vi "水样测试.vi"(11 "数据标记表":string(combo)="N") -> ()   [LabVIEW 2016, in "斯坦道多参数.lvlib"]
panel:
  out "运行状态":u16(ring) items=["空闲", "水样测试", "标样核查"]
  out "多参数运行日志":string
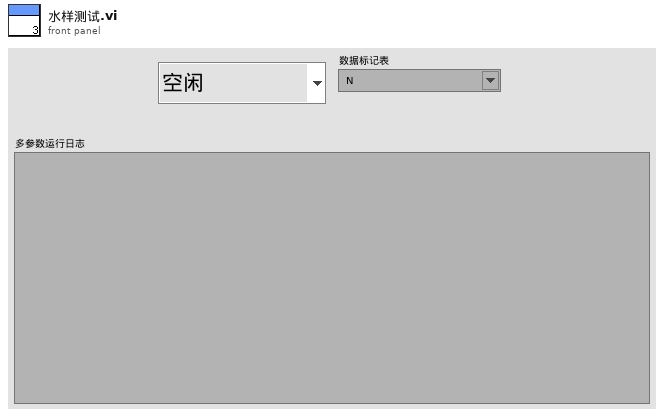
[diagram p1: front panel]
types:
  T1 = typedef "集成多参数单参数字段定义.ctl" = cluster{"时间":timestamp, "测量模式":string, "数据类型":string, "检测值":sgl, "单位":string, "数据标识":string, "信号值":sgl, "标样参考值":sgl, "因子编码":string, "探头温度":sgl, "LastTime":timestamp}
  T2 = cluster{"水温":bool, "pH":bool, "DO":bool, "DOper":bool, "电导率":bool, "ORP":bool, "浊度":bool, "叶绿素a":bool, "藻密度":bool, "COD":bool, "DO2":bool, "DOper":bool, "氯化物":bool, "氨氮":bool, "水中油":bool, "悬浮物":bool, "余氯":bool}
  T3 = cluster{"ph":bool, "DO":bool, "Cond":bool, "Turb":bool, "叶绿素a":bool, "藻密度":bool, "ORP":bool, "cod":bool, "DO2":bool, "氯化物":bool, "氨氮":bool, "水中油":bool, "悬浮物":bool, "余氯":bool}
  T4 = cluster{"温度测量值":sgl, "测量值":sgl, "温度偏移修正值":sgl, "信号值":sgl, "数据标识":string}
  T5 = cluster{"温度测量值":sgl, "DO%":sgl, "DOmg/L":sgl, "温度偏移修正值":sgl, "数据标识mg/L":string, "数据标识%":string}
  T6 = cluster{"CH":u16, "监测值":dbl, "信号值":sgl, "数据标识":string}
  T7 = cluster{"水样数据时间":timestamp, "水温":dbl, "pH":dbl, "DO":dbl, "DOper":dbl, "电导率":dbl, "ORP":dbl, "浊度":dbl, "叶绿素a":dbl, "藻密度":dbl, "COD":dbl, "DO2":dbl, "DO2per":dbl, "氯化物":dbl, "氨氮":dbl, "水中油":dbl, "悬浮物":dbl, "余氯":dbl}
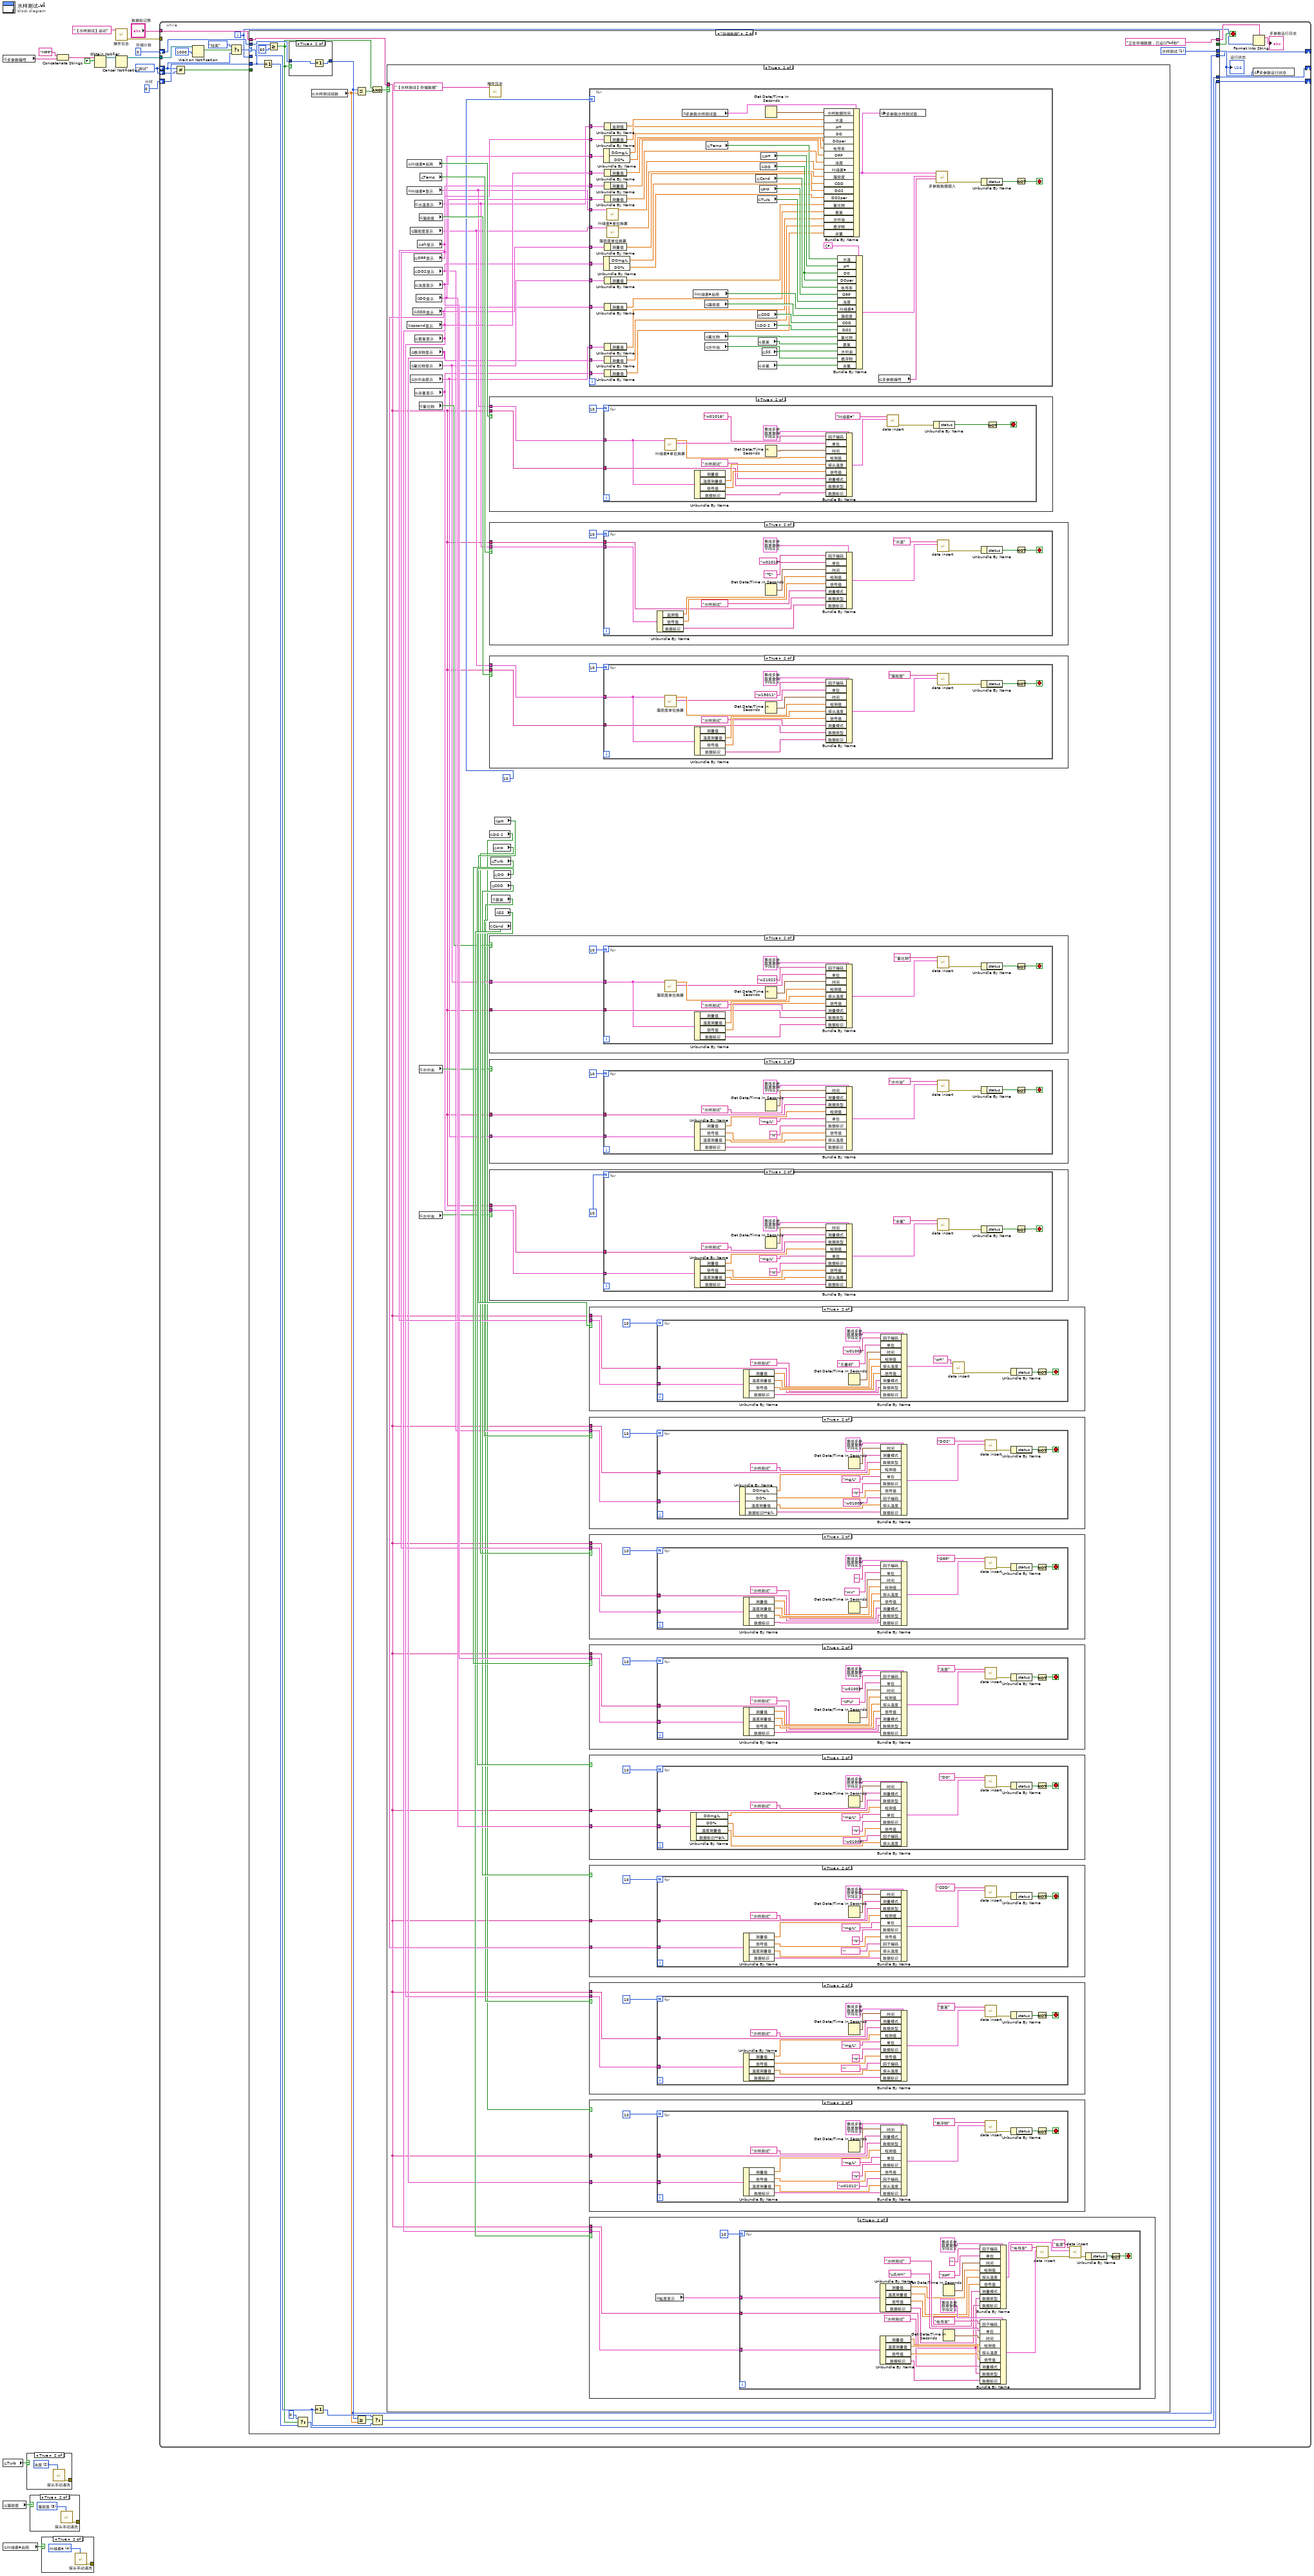
[diagram p0: block diagram]
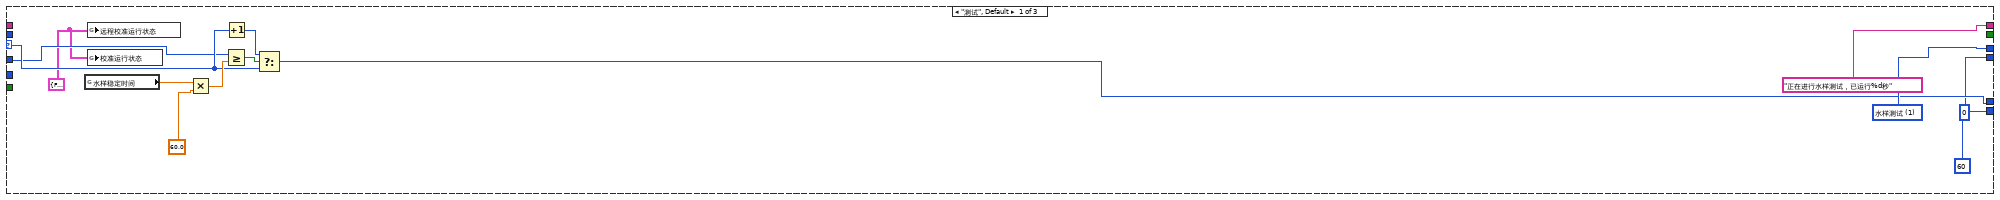
[diagram p5: hidden frame]
diagram:
  w7 = 0  # 存储计数
  w8 = 0  # 计时
  w3 = enum16{"测试", "存储数据", "结束"}."测试" ("枚举")
  n1 = global read "多参数全局变量.vi" "多参数编号"() -> (w9:string)
  n2 = global read "断电保存变量.vi" "Turb"() -> (w6:bool)
  n3 = global read "断电保存变量.vi" "藻密度"() -> (w4:bool)
  n4 = global read "断电保存变量.vi" "叶绿素a启用"() -> (w5:bool)
  n5 = case shown="True" w6 {
    tunnel: [_ w16] -> _
    frame False {
    }
    frame True {
      w17 = u16 2 items=["pH", "DO", "浊度", "电导率", "叶绿素a", "藻密度", "ORP", "DO2"] ("校准参数")
      n6 = call "探头手动清洗.vi"("校准参数"=w17) -> ("error out"=w16:errorcluster)  [unwired: 10 in]
    }
  }
  n7 = case shown="True" w4 {
    tunnel: [_ w18] -> _
    frame False {
    }
    frame True {
      w19 = u16 5 items=["pH", "DO", "浊度", "电导率", "叶绿素a", "藻密度", "ORP", "DO2"] ("校准参数")
      n8 = call "探头手动清洗.vi"("校准参数"=w19) -> ("error out"=w18:errorcluster)  [unwired: 10 in]
    }
  }
  n9 = case shown="True" w5 {
    tunnel: [_ w20] -> _
    frame False {
    }
    frame True {
      w21 = u16 4 items=["pH", "DO", "浊度", "电导率", "叶绿素a", "藻密度", "ORP", "DO2"] ("校准参数")
      n10 = call "探头手动清洗.vi"("校准参数"=w21) -> ("error out"=w20:errorcluster)  [unwired: 10 in]
    }
  }
  n11 = Concatenate Strings("MPP" ("名称（未命名）"), w9) -> (w10:string)
  n12 = Obtain Notifier(name (unnamed)=w10, notification data type=FALSE) -> (notifier out=w13:refnum<notifier>)  [unwired: 2 in, 2 out]
  n13 = call "操作日志.vi"("日志信息"="【水样测试】启动") -> ("error out"=w1:errorcluster)  [unwired: 10 in]
  n14 = Cancel Notification(0:w13) -> (8:w12:refnum<notifier>)  [unwired: 1 in, 2 out]
  n15 = while {
    shift-right: [w26] -> _
    shift-left: w3 -> [w24]
    tunnel: w12 -> [w37]
    tunnel: "数据标记表" -> [w32]
    shift-right: [w28] -> _
    shift-left: w8 -> [w30]
    shift-right: [w27] -> _
    shift-left: w7 -> [w29]
    shift-left: w3 -> [w23]
    tunnel: w1 -> [_]
    i -> [w25]
    stop <- w40 stop-if-true
    n16 = Not Equal?(x=w24, y=w23) -> (x != y?=w22:bool)
    n17 = Wait on Notification(notifier=w37, timeout in ms (-1)=1000 ("超时毫秒(-1)")) -> (notification=w35:bool)  [unwired: 2 in, 3 out]
    n18 = Select(t=enum16{"测试", "存储数据", "结束"}."结束" ("枚举"), s=w35, f=w24) -> (s? t:f=w33:enum16{"测试", "存储数据", "结束"})
    n19 = case shown="\"存储数据\"" w33 {
      selector: w33 -> [w47 w61 _]
      tunnel: [_ _ TRUE] -> w40
      tunnel: ["正在进行水样测试，已运行%d秒" ("格式字符串") "正在存储数据，已运行%d秒" ("格式字符串") "测试停止，累计运行%d秒" ("格式字符串")] -> w39
      tunnel: [w52 w66 w470] -> w31
      tunnel: w32 -> [_ w71 _]
      tunnel: w30 -> [_ w69 _]
      tunnel: w29 -> [_ w70 _]
      tunnel: [60 w54 0] -> w28
      tunnel: [0 w60 0] -> w27
      tunnel: [w45 w64 enum16{"测试", "存储数据", "结束"}."结束" ("枚举")] -> w26
      tunnel: w25 -> [w42 _ _]
      tunnel: w22 -> [_ _ w466]
      frame "测试", Default {
        w41 = T3 {"ph"=FALSE, "DO"=FALSE, "Cond"=FALSE, "Turb"=FALSE, "叶绿素a"=FALSE, "藻密度"=FALSE, "ORP"=FALSE, "cod"=FALSE, "DO2"=FALSE, "氯化物"=FALSE, "氨氮"=FALSE, "水中油"=FALSE, "悬浮物"=FALSE, "余氯"=FALSE} ("远程校准运行状态")
        w52 = u16 1 items=["空闲", "水样测试", "标样核查"] ("多参数运行状态")
        n20 = global read "断电保存变量.vi" "水样稳定时间"() -> (w51:dbl)
        n21 = global write "多参数全局变量.vi" "远程校准运行状态"(w41) -> ()
        n22 = global write "多参数全局变量.vi" "校准运行状态"(w41) -> ()
        n23 = Multiply(x=w51, y=60.0) -> (x*y=w49:dbl)
        n24 = Greater Or Equal?(x=w42, y=w49) -> (x >= y?=w48:bool)
        n25 = Increment(x=w47) -> (x+1=w46:enum16{"测试", "存储数据", "结束"})
        n26 = Select(t=w46, s=w48, f=w47) -> (s? t:f=w45:enum16{"测试", "存储数据", "结束"})
      }
      frame "存储数据" {
        w66 = u16 1 items=["空闲", "水样测试", "标样核查"] ("多参数运行状态")
        n27 = Increment(x=w69) -> (x+1=w56:i32)
        n28 = Greater Or Equal?(x=w69, y=60) -> (x >= y?=w57:bool)
        n29 = case shown="True" w57 {
          tunnel: w70 -> [w72 w74]
          tunnel: [w72 w73] -> w60
          frame False {
          }
          frame True {
            n30 = Increment(x=w74) -> (x+1=w73:i32)
          }
        }
        n31 = Select(t=0, s=w57, f=w56) -> (s? t:f=w54:i32)
        n32 = global read "断电保存变量.vi" "水样测试组数"() -> (w59:dbl)
        n33 = Increment(x=w61) -> (x+1=w62:enum16{"测试", "存储数据", "结束"})
        n34 = Less Or Equal?(x=w60, y=w59) -> (x <= y?=w65:bool)
        n35 = Greater Or Equal?(x=w60, y=w59) -> (x >= y?=w58:bool)
        n36 = And(x=w57, y=w65) -> (x .and. y?=w63:bool)
        n37 = Select(t=w62, s=w58, f=w61) -> (s? t:f=w64:enum16{"测试", "存储数据", "结束"})
        n38 = case shown="True" w63 {
          tunnel: w71 -> [_ w75]
          frame False {
          }
          frame True {
            n39 = global read "断电保存变量.vi" "叶绿素a启用"() -> (w107:bool)
            n40 = global read "多参数全局变量.vi" "叶绿素a显示"() -> (w92:T4)
            n41 = global read "多参数全局变量.vi" "spcond显示"() -> (w98:T4)
            n42 = global read "多参数全局变量.vi" "藻密度显示"() -> (w94:T4)
            n43 = global read "多参数全局变量.vi" "悬浮物显示"() -> (w79:T4)
            n44 = global read "多参数全局变量.vi" "氯化物显示"() -> (w84:T4)
            n45 = global read "多参数全局变量.vi" "水中油显示"() -> (w80:T4)
            n46 = global read "多参数全局变量.vi" "COD显示"() -> (w89:T4)
            n47 = global read "多参数全局变量.vi" "ORP显示"() -> (w91:T4)
            n48 = global read "多参数全局变量.vi" "DO2显示"() -> (w86:T5)
            n49 = global read "多参数全局变量.vi" "水温显示"() -> (w93:T6)
            n50 = global read "多参数全局变量.vi" "浊度显示"() -> (w96:T4)
            n51 = global read "多参数全局变量.vi" "氨氮显示"() -> (w82:T4)
            n52 = global read "多参数全局变量.vi" "余氯显示"() -> (w76:T4)
            n53 = global read "多参数全局变量.vi" "DO显示"() -> (w95:T5)
            n54 = global read "多参数全局变量.vi" "ph显示"() -> (w97:T4)
            n55 = global read "断电保存变量.vi" "藻密度"() -> (w101:bool)
            n56 = global read "断电保存变量.vi" "氯化物"() -> (w85:bool)
            n57 = global read "断电保存变量.vi" "水中油"() -> (w81:bool)
            n58 = global read "断电保存变量.vi" "水中油"() -> (w77:bool)
            n59 = global read "断电保存变量.vi" "Temp"() -> (w102:bool)
            n60 = call "操作日志.vi"("日志信息"="【水样测试】存储数据") -> ()  [unwired: 10 in, 1 out]
            n61 = case shown="True" w107 {
              tunnel: w75 -> [_ w341]
              tunnel: w92 -> [_ w339]
              frame False {
              }
              frame True {
                n62 = for {
                  N: 10 -> [_]
                  tunnel: w341 -> [w347]
                  tunnel: w339 -> [w344]
                  stop <- w351 stop-if-true
                  n63 = call "叶绿素a单位换算.vi"("叶绿素a显示"=w344) -> ("检测值1.单位"=w343:string, "测量值"=w342:sgl)  [unwired: 8 in, 1 out]
                  n64 = Unbundle By Name(w344) -> ("温度测量值"=w357:sgl, "信号值"=w350:sgl, "数据标识"=w346:string)  [unwired: 1 out]
                  n65 = Get Date/Time In Seconds() -> (seconds since 1Jan1904=w349:timestamp)
                  n66 = Bundle By Name(cluster=T1 {"时间"=timestamp(0 s since 1904-01-01), "测量模式"="水样测试", "数据类型"="N", "检测值"=0.0, "单位"="mg/L", "数据标识"="N", "信号值"=0.0, "标样参考值"=0.0, "因子编码"="", "探头温度"=0.0, "LastTime"=timestamp(0 s since 1904-01-01)} ("data"), "因子编码"="w01016", "单位"=w343, "时间"=w349, "检测值"=w342, "探头温度"=w357, "信号值"=w350, "测量模式"="水样测试", "数据类型"=w347, "数据标识"=w346) -> (w355:T1)
                  n67 = call "data insert.vi"("data"=w355, "table in"="叶绿素a" ("table输入")) -> ("error out"=w353:errorcluster)  [unwired: 9 in]
                  n68 = Unbundle By Name(w353) -> ("status"=w352:bool)
                  n69 = Not(x=w352) -> (.not. x?=w351:bool)
                }
              }
            }
            n70 = case shown="True" w102 {
              tunnel: w75 -> [_ w450]
              tunnel: w93 -> [_ w448]
              frame False {
              }
              frame True {
                n71 = for {
                  N: 10 -> [_]
                  tunnel: w450 -> [w454]
                  tunnel: w448 -> [w453]
                  stop <- w458 stop-if-true
                  n72 = Unbundle By Name(w453) -> ("监测值"=w461:dbl, "信号值"=w456:sgl, "数据标识"=w452:string)
                  n73 = Get Date/Time In Seconds() -> (seconds since 1Jan1904=w457:timestamp)
                  n74 = Bundle By Name(cluster=T1 {"时间"=timestamp(0 s since 1904-01-01), "测量模式"="水样测试", "数据类型"="N", "检测值"=0.0, "单位"="mg/L", "数据标识"="N", "信号值"=0.0, "标样参考值"=0.0, "因子编码"="", "探头温度"=0.0, "LastTime"=timestamp(0 s since 1904-01-01)} ("data"), "因子编码"="w01010", "单位"="℃", "时间"=w457, "检测值"=w461, "信号值"=w456, "测量模式"="水样测试", "数据类型"=w454, "数据标识"=w452) -> (w464:T1)
                  n75 = call "data insert.vi"("data"=w464, "table in"="水温" ("table输入")) -> ("error out"=w460:errorcluster)  [unwired: 9 in]
                  n76 = Unbundle By Name(w460) -> ("status"=w459:bool)
                  n77 = Not(x=w459) -> (.not. x?=w458:bool)
                }
              }
            }
            n78 = case shown="True" w101 {
              tunnel: w75 -> [_ w322]
              tunnel: w94 -> [_ w320]
              frame False {
              }
              frame True {
                n79 = for {
                  N: 10 -> [_]
                  tunnel: w322 -> [w329]
                  tunnel: w320 -> [w325]
                  stop <- w330 stop-if-true
                  n80 = call "藻密度单位换算.vi"("藻密度显示"=w325) -> ("检测值1.单位"=w323:string, "测量值"=w324:sgl)  [unwired: 8 in, 1 out]
                  n81 = Unbundle By Name(w325) -> ("温度测量值"=w338:sgl, "信号值"=w331:sgl, "数据标识"=w327:string)  [unwired: 1 out]
                  n82 = Get Date/Time In Seconds() -> (seconds since 1Jan1904=w332:timestamp)
                  n83 = Bundle By Name(cluster=T1 {"时间"=timestamp(0 s since 1904-01-01), "测量模式"="水样测试", "数据类型"="N", "检测值"=0.0, "单位"="mg/L", "数据标识"="N", "信号值"=0.0, "标样参考值"=0.0, "因子编码"="", "探头温度"=0.0, "LastTime"=timestamp(0 s since 1904-01-01)} ("data"), "因子编码"="w19011", "单位"=w323, "时间"=w332, "检测值"=w324, "探头温度"=w338, "信号值"=w331, "测量模式"="水样测试", "数据类型"=w329, "数据标识"=w327) -> (w333:T1)
                  n84 = call "data insert.vi"("data"=w333, "table in"="藻密度" ("table输入")) -> ("error out"=w335:errorcluster)  [unwired: 9 in]
                  n85 = Unbundle By Name(w335) -> ("status"=w334:bool)
                  n86 = Not(x=w334) -> (.not. x?=w330:bool)
                }
              }
            }
            n87 = global read "断电保存变量.vi" "DO 2"() -> (w87:bool)
            n88 = global read "断电保存变量.vi" "Cond"() -> (w105:bool)
            n89 = case shown="True" w85 {
              tunnel: w75 -> [_ w188]
              tunnel: w84 -> [_ w186]
              frame False {
              }
              frame True {
                n90 = for {
                  N: 10 -> [_]
                  tunnel: w188 -> [w197]
                  tunnel: w186 -> [w193]
                  stop <- w198 stop-if-true
                  n91 = call "藻密度单位换算.vi"("藻密度显示"=w193) -> ("检测值1.单位"=w191:string, "测量值"=w192:sgl)  [unwired: 8 in, 1 out]
                  n92 = Unbundle By Name(w193) -> ("温度测量值"=w204:sgl, "信号值"=w199:sgl, "数据标识"=w195:string)  [unwired: 1 out]
                  n93 = Get Date/Time In Seconds() -> (seconds since 1Jan1904=w200:timestamp)
                  n94 = Bundle By Name(cluster=T1 {"时间"=timestamp(0 s since 1904-01-01), "测量模式"="水样测试", "数据类型"="N", "检测值"=0.0, "单位"="mg/L", "数据标识"="N", "信号值"=0.0, "标样参考值"=0.0, "因子编码"="", "探头温度"=0.0, "LastTime"=timestamp(0 s since 1904-01-01)} ("data"), "因子编码"="w21022", "单位"=w191, "时间"=w200, "检测值"=w192, "探头温度"=w204, "信号值"=w199, "测量模式"="水样测试", "数据类型"=w197, "数据标识"=w195) -> (w201:T1)
                  n95 = call "data insert.vi"("data"=w201, "table in"="氯化物") -> ("error out"=w203:errorcluster)  [unwired: 9 in]
                  n96 = Unbundle By Name(w203) -> ("status"=w202:bool)
                  n97 = Not(x=w202) -> (.not. x?=w198:bool)
                }
              }
            }
            n98 = case shown="True" w81 {
              tunnel: w75 -> [_ w149]
              tunnel: w80 -> [_ w147]
              frame False {
              }
              frame True {
                n99 = for {
                  N: 10 -> [_]
                  tunnel: w149 -> [w162]
                  tunnel: w147 -> [w155]
                  stop <- w165 stop-if-true
                  n100 = Unbundle By Name(w155) -> ("测量值"=w154:sgl, "信号值"=w153:sgl, "温度测量值"=w152:sgl, "数据标识"=w151:string)
                  n101 = Get Date/Time In Seconds() -> (seconds since 1Jan1904=w164:timestamp)
                  n102 = Bundle By Name(cluster=T1 {"时间"=timestamp(0 s since 1904-01-01), "测量模式"="水样测试", "数据类型"="N", "检测值"=0.0, "单位"="mg/L", "数据标识"="N", "信号值"=0.0, "标样参考值"=0.0, "因子编码"="", "探头温度"=0.0, "LastTime"=timestamp(0 s since 1904-01-01)} ("data"), "时间"=w164, "测量模式"="水样测试", "数据类型"=w162, "检测值"=w154, "单位"="mg/L", "数据标识"="N" ("水样数据标识"), "信号值"=w153, "探头温度"=w152, "数据标识"=w151) -> (w157:T1)
                  n103 = call "data insert.vi"("data"=w157, "table in"="水中油") -> ("error out"=w158:errorcluster)  [unwired: 9 in]
                  n104 = Unbundle By Name(w158) -> ("status"=w159:bool)
                  n105 = Not(x=w159) -> (.not. x?=w165:bool)
                }
              }
            }
            n106 = case shown="True" w77 {
              tunnel: w75 -> [_ w110]
              tunnel: w76 -> [_ w108]
              frame False {
              }
              frame True {
                n107 = for {
                  N: 10 -> [_]
                  tunnel: w110 -> [w123]
                  tunnel: w108 -> [w116]
                  stop <- w126 stop-if-true
                  n108 = Unbundle By Name(w116) -> ("测量值"=w115:sgl, "信号值"=w114:sgl, "温度测量值"=w113:sgl, "数据标识"=w112:string)
                  n109 = Get Date/Time In Seconds() -> (seconds since 1Jan1904=w125:timestamp)
                  n110 = Bundle By Name(cluster=T1 {"时间"=timestamp(0 s since 1904-01-01), "测量模式"="水样测试", "数据类型"="N", "检测值"=0.0, "单位"="mg/L", "数据标识"="N", "信号值"=0.0, "标样参考值"=0.0, "因子编码"="", "探头温度"=0.0, "LastTime"=timestamp(0 s since 1904-01-01)} ("data"), "时间"=w125, "测量模式"="水样测试", "数据类型"=w123, "检测值"=w115, "单位"="mg/L", "数据标识"="N" ("水样数据标识"), "信号值"=w114, "探头温度"=w113, "数据标识"=w112) -> (w118:T1)
                  n111 = call "data insert.vi"("data"=w118, "table in"="余氯") -> ("error out"=w119:errorcluster)  [unwired: 9 in]
                  n112 = Unbundle By Name(w119) -> ("status"=w120:bool)
                  n113 = Not(x=w120) -> (.not. x?=w126:bool)
                }
              }
            }
            n114 = global read "断电保存变量.vi" "Turb"() -> (w106:bool)
            n115 = global read "断电保存变量.vi" "COD"() -> (w88:bool)
            n116 = global read "断电保存变量.vi" "氨氮"() -> (w83:bool)
            n117 = global read "断电保存变量.vi" "orp"() -> (w100:bool)
            n118 = global read "断电保存变量.vi" "DO"() -> (w104:bool)
            n119 = global read "断电保存变量.vi" "pH"() -> (w103:bool)
            n120 = global read "断电保存变量.vi" "SS"() -> (w78:bool)
            n121 = for {
              N: 10 -> [_]
              tunnel: w93 -> [w280]
              tunnel: w97 -> [w279]
              tunnel: w95 -> [w278]
              tunnel: w98 -> [w277]
              tunnel: w91 -> [w276]
              tunnel: w96 -> [w275]
              tunnel: w92 -> [w265]
              tunnel: w94 -> [w267]
              tunnel: w89 -> [w273]
              tunnel: w86 -> [w270]
              tunnel: w84 -> [w261]
              tunnel: w82 -> [w259]
              tunnel: w80 -> [w252]
              tunnel: w79 -> [w249]
              tunnel: w76 -> [w246]
              stop <- w282 stop-if-true
              n122 = Unbundle By Name(w278) -> ("DOmg/L"=w297:sgl, "DO%"=w296:sgl)
              n123 = Unbundle By Name(w270) -> ("DOmg/L"=w269:sgl, "DO%"=w268:sgl)
              n124 = Unbundle By Name(w280) -> ("监测值"=w299:dbl)
              n125 = Unbundle By Name(w279) -> ("测量值"=w298:sgl)
              n126 = Unbundle By Name(w277) -> ("测量值"=w295:sgl)
              n127 = Unbundle By Name(w276) -> ("测量值"=w294:sgl)
              n128 = Unbundle By Name(w275) -> ("测量值"=w293:sgl)
              n129 = Unbundle By Name(w273) -> ("测量值"=w272:sgl)
              n130 = Unbundle By Name(w261) -> ("测量值"=w260:sgl)
              n131 = Unbundle By Name(w259) -> ("测量值"=w258:sgl)
              n132 = Unbundle By Name(w252) -> ("测量值"=w251:sgl)
              n133 = Unbundle By Name(w249) -> ("测量值"=w248:sgl)
              n134 = Unbundle By Name(w246) -> ("测量值"=w245:sgl)
              n135 = call "叶绿素a单位换算.vi"("叶绿素a显示"=w265) -> ("测量值"=w264:sgl)  [unwired: 8 in, 2 out]
              n136 = call "藻密度单位换算.vi"("藻密度显示"=w267) -> ("测量值"=w266:sgl)  [unwired: 8 in, 2 out]
              n137 = global read "多参数全局变量.vi" "多参数水样测试值"() -> (w256:T7)
              n138 = global read "断电保存变量.vi" "叶绿素a启用"() -> (w286:bool)
              n139 = global read "断电保存变量.vi" "藻密度"() -> (w289:bool)
              n140 = global read "断电保存变量.vi" "氯化物"() -> (w262:bool)
              n141 = global read "断电保存变量.vi" "水中油"() -> (w253:bool)
              n142 = global read "断电保存变量.vi" "Temp"() -> (w288:bool)
              n143 = global read "断电保存变量.vi" "Cond"() -> (w291:bool)
              n144 = global read "断电保存变量.vi" "DO 2"() -> (w271:bool)
              n145 = global read "断电保存变量.vi" "Turb"() -> (w290:bool)
              n146 = global read "断电保存变量.vi" "COD"() -> (w274:bool)
              n147 = global read "断电保存变量.vi" "氨氮"() -> (w257:bool)
              n148 = global read "断电保存变量.vi" "余氯"() -> (w247:bool)
              n149 = global read "断电保存变量.vi" "orp"() -> (w287:bool)
              n150 = global read "断电保存变量.vi" "DO"() -> (w285:bool)
              n151 = global read "断电保存变量.vi" "pH"() -> (w292:bool)
              n152 = global read "断电保存变量.vi" "SS"() -> (w250:bool)
              n153 = Get Date/Time In Seconds() -> (seconds since 1Jan1904=w300:timestamp)
              n154 = Bundle By Name(cluster=w256, "水样数据时间"=w300, "水温"=w299, "pH"=w298, "DO"=w297, "DOper"=w296, "电导率"=w295, "ORP"=w294, "浊度"=w293, "叶绿素a"=w264, "藻密度"=w266, "COD"=w272, "DO2"=w269, "DO2per"=w268, "氯化物"=w260, "氨氮"=w258, "水中油"=w251, "悬浮物"=w248, "余氯"=w245) -> (w263:T7)
              n155 = Bundle By Name(cluster=T2 {"水温"=FALSE, "pH"=FALSE, "DO"=FALSE, "DOper"=FALSE, "电导率"=FALSE, "ORP"=FALSE, "浊度"=FALSE, "叶绿素a"=FALSE, "藻密度"=FALSE, "COD"=FALSE, "DO2"=FALSE, "DOper"=FALSE, "氯化物"=FALSE, "氨氮"=FALSE, "水中油"=FALSE, "悬浮物"=FALSE, "余氯"=FALSE} ("columns enable"), "水温"=w288, "pH"=w292, "DO"=w285, "DOper"=w285, "电导率"=w291, "ORP"=w287, "浊度"=w290, "叶绿素a"=w286, "藻密度"=w289, "COD"=w274, "DO2"=w271, "氯化物"=w262, "氨氮"=w257, "水中油"=w253, "悬浮物"=w250, "余氯"=w247) -> (w254:T2)
              n156 = global read "多参数全局变量.vi" "多参数编号"() -> (w281:string)
              n157 = global write "多参数全局变量.vi" "多参数水样测试值"(w263) -> ()
              n158 = call "多参数数据插入.vi"("编号"=w281, "columns enable"=w254, "data in"=w263) -> ("error out"=w284:errorcluster)  [unwired: 8 in]
              n159 = Unbundle By Name(w284) -> ("status"=w283:bool)
              n160 = Not(x=w283) -> (.not. x?=w282:bool)
            }
            n161 = case shown="True" w103 {
              tunnel: w75 -> [_ w431]
              tunnel: w97 -> [_ w429]
              frame False {
              }
              frame True {
                n162 = for {
                  N: 10 -> [_]
                  tunnel: w431 -> [w435]
                  tunnel: w429 -> [w434]
                  stop <- w439 stop-if-true
                  n163 = Unbundle By Name(w434) -> ("测量值"=w443:sgl, "温度测量值"=w442:sgl, "信号值"=w437:sgl, "数据标识"=w433:string)
                  n164 = Get Date/Time In Seconds() -> (seconds since 1Jan1904=w438:timestamp)
                  n165 = Bundle By Name(cluster=T1 {"时间"=timestamp(0 s since 1904-01-01), "测量模式"="水样测试", "数据类型"="N", "检测值"=0.0, "单位"="mg/L", "数据标识"="N", "信号值"=0.0, "标样参考值"=0.0, "因子编码"="", "探头温度"=0.0, "LastTime"=timestamp(0 s since 1904-01-01)} ("data"), "因子编码"="w01001", "单位"="无量纲", "时间"=w438, "检测值"=w443, "探头温度"=w442, "信号值"=w437, "测量模式"="水样测试", "数据类型"=w435, "数据标识"=w433) -> (w447:T1)
                  n166 = call "data insert.vi"("data"=w447, "table in"="pH" ("table输入")) -> ("error out"=w441:errorcluster)  [unwired: 9 in]
                  n167 = Unbundle By Name(w441) -> ("status"=w440:bool)
                  n168 = Not(x=w440) -> (.not. x?=w439:bool)
                }
              }
            }
            n169 = case shown="True" w87 {
              tunnel: w75 -> [_ w207]
              tunnel: w86 -> [_ w205]
              frame False {
              }
              frame True {
                n170 = for {
                  N: 10 -> [_]
                  tunnel: w207 -> [w221]
                  tunnel: w205 -> [w211]
                  stop <- w224 stop-if-true
                  n171 = Unbundle By Name(w211) -> ("DOmg/L"=w220:sgl, "DO%"=w213:sgl, "温度测量值"=w214:sgl, "数据标识mg/L"=w210:string)
                  n172 = Get Date/Time In Seconds() -> (seconds since 1Jan1904=w223:timestamp)
                  n173 = Bundle By Name(cluster=T1 {"时间"=timestamp(0 s since 1904-01-01), "测量模式"="水样测试", "数据类型"="N", "检测值"=0.0, "单位"="mg/L", "数据标识"="N", "信号值"=0.0, "标样参考值"=0.0, "因子编码"="", "探头温度"=0.0, "LastTime"=timestamp(0 s since 1904-01-01)} ("data"), "时间"=w223, "测量模式"="水样测试", "数据类型"=w221, "检测值"=w220, "单位"="mg/L", "数据标识"="N" ("水样数据标识"), "信号值"=w213, "因子编码"="w01009", "探头温度"=w214, "数据标识"=w210) -> (w212:T1)
                  n174 = call "data insert.vi"("data"=w212, "table in"="DO2") -> ("error out"=w216:errorcluster)  [unwired: 9 in]
                  n175 = Unbundle By Name(w216) -> ("status"=w217:bool)
                  n176 = Not(x=w217) -> (.not. x?=w224:bool)
                }
              }
            }
            n177 = case shown="True" w100 {
              tunnel: w75 -> [_ w303]
              tunnel: w91 -> [_ w301]
              frame False {
              }
              frame True {
                n178 = for {
                  N: 10 -> [_]
                  tunnel: w303 -> [w309]
                  tunnel: w301 -> [w307]
                  stop <- w312 stop-if-true
                  n179 = Unbundle By Name(w307) -> ("测量值"=w319:sgl, "温度测量值"=w317:sgl, "信号值"=w310:sgl, "数据标识"=w306:string)
                  n180 = Get Date/Time In Seconds() -> (seconds since 1Jan1904=w311:timestamp)
                  n181 = Bundle By Name(cluster=T1 {"时间"=timestamp(0 s since 1904-01-01), "测量模式"="水样测试", "数据类型"="N", "检测值"=0.0, "单位"="mg/L", "数据标识"="N", "信号值"=0.0, "标样参考值"=0.0, "因子编码"="", "探头温度"=0.0, "LastTime"=timestamp(0 s since 1904-01-01)} ("data"), "因子编码"="", "单位"="mV", "时间"=w311, "检测值"=w319, "探头温度"=w317, "信号值"=w310, "测量模式"="水样测试", "数据类型"=w309, "数据标识"=w306) -> (w304:T1)
                  n182 = call "data insert.vi"("data"=w304, "table in"="ORP" ("table输入")) -> ("error out"=w315:errorcluster)  [unwired: 9 in]
                  n183 = Unbundle By Name(w315) -> ("status"=w314:bool)
                  n184 = Not(x=w314) -> (.not. x?=w312:bool)
                }
              }
            }
            n185 = case shown="True" w106 {
              tunnel: w75 -> [_ w360]
              tunnel: w96 -> [_ w358]
              frame False {
              }
              frame True {
                n186 = for {
                  N: 10 -> [_]
                  tunnel: w360 -> [w364]
                  tunnel: w358 -> [w363]
                  stop <- w368 stop-if-true
                  n187 = Unbundle By Name(w363) -> ("测量值"=w372:sgl, "温度测量值"=w371:sgl, "信号值"=w366:sgl, "数据标识"=w362:string)
                  n188 = Get Date/Time In Seconds() -> (seconds since 1Jan1904=w367:timestamp)
                  n189 = Bundle By Name(cluster=T1 {"时间"=timestamp(0 s since 1904-01-01), "测量模式"="水样测试", "数据类型"="N", "检测值"=0.0, "单位"="mg/L", "数据标识"="N", "信号值"=0.0, "标样参考值"=0.0, "因子编码"="", "探头温度"=0.0, "LastTime"=timestamp(0 s since 1904-01-01)} ("data"), "因子编码"="w01003", "单位"="NTU", "时间"=w367, "检测值"=w372, "探头温度"=w371, "信号值"=w366, "测量模式"="水样测试", "数据类型"=w364, "数据标识"=w362) -> (w375:T1)
                  n190 = call "data insert.vi"("data"=w375, "table in"="浊度" ("table输入")) -> ("error out"=w370:errorcluster)  [unwired: 9 in]
                  n191 = Unbundle By Name(w370) -> ("status"=w369:bool)
                  n192 = Not(x=w369) -> (.not. x?=w368:bool)
                }
              }
            }
            n193 = case shown="True" w104 {
              tunnel: w75 -> [_ w412]
              tunnel: w95 -> [_ w410]
              frame False {
              }
              frame True {
                n194 = for {
                  N: 10 -> [_]
                  tunnel: w412 -> [w424]
                  tunnel: w410 -> [w415]
                  stop <- w428 stop-if-true
                  n195 = Unbundle By Name(w415) -> ("DOmg/L"=w423:sgl, "DO%"=w417:sgl, "温度测量值"=w418:sgl)  [unwired: 1 out]
                  n196 = Get Date/Time In Seconds() -> (seconds since 1Jan1904=w426:timestamp)
                  n197 = Bundle By Name(cluster=T1 {"时间"=timestamp(0 s since 1904-01-01), "测量模式"="水样测试", "数据类型"="N", "检测值"=0.0, "单位"="mg/L", "数据标识"="N", "信号值"=0.0, "标样参考值"=0.0, "因子编码"="", "探头温度"=0.0, "LastTime"=timestamp(0 s since 1904-01-01)} ("data"), "时间"=w426, "测量模式"="水样测试", "数据类型"=w424, "检测值"=w423, "单位"="mg/L", "数据标识"="N", "信号值"=w417, "因子编码"="w01009", "探头温度"=w418) -> (w416:T1)
                  n198 = call "data insert.vi"("data"=w416, "table in"="DO") -> ("error out"=w420:errorcluster)  [unwired: 9 in]
                  n199 = Unbundle By Name(w420) -> ("status"=w421:bool)
                  n200 = Not(x=w421) -> (.not. x?=w428:bool)
                }
              }
            }
            n201 = case shown="True" w88 {
              tunnel: w75 -> [_ w227]
              tunnel: w89 -> [_ w225]
              frame False {
              }
              frame True {
                n202 = for {
                  N: 10 -> [_]
                  tunnel: w227 -> [w240]
                  tunnel: w225 -> [w230]
                  stop <- w244 stop-if-true
                  n203 = Unbundle By Name(w230) -> ("测量值"=w239:sgl, "信号值"=w232:sgl, "温度测量值"=w233:sgl, "数据标识"=w229:string)
                  n204 = Get Date/Time In Seconds() -> (seconds since 1Jan1904=w242:timestamp)
                  n205 = Bundle By Name(cluster=T1 {"时间"=timestamp(0 s since 1904-01-01), "测量模式"="水样测试", "数据类型"="N", "检测值"=0.0, "单位"="mg/L", "数据标识"="N", "信号值"=0.0, "标样参考值"=0.0, "因子编码"="", "探头温度"=0.0, "LastTime"=timestamp(0 s since 1904-01-01)} ("data"), "时间"=w242, "测量模式"="水样测试", "数据类型"=w240, "检测值"=w239, "单位"="mg/L", "数据标识"="N" ("水样数据标识"), "信号值"=w232, "因子编码"="", "探头温度"=w233, "数据标识"=w229) -> (w231:T1)
                  n206 = call "data insert.vi"("data"=w231, "table in"="COD") -> ("error out"=w235:errorcluster)  [unwired: 9 in]
                  n207 = Unbundle By Name(w235) -> ("status"=w236:bool)
                  n208 = Not(x=w236) -> (.not. x?=w244:bool)
                }
              }
            }
            n209 = case shown="True" w83 {
              tunnel: w75 -> [_ w168]
              tunnel: w82 -> [_ w166]
              frame False {
              }
              frame True {
                n210 = for {
                  N: 10 -> [_]
                  tunnel: w168 -> [w181]
                  tunnel: w166 -> [w173]
                  stop <- w185 stop-if-true
                  n211 = Unbundle By Name(w173) -> ("测量值"=w172:sgl, "信号值"=w171:sgl, "温度测量值"=w170:sgl, "数据标识"=w169:string)
                  n212 = Get Date/Time In Seconds() -> (seconds since 1Jan1904=w183:timestamp)
                  n213 = Bundle By Name(cluster=T1 {"时间"=timestamp(0 s since 1904-01-01), "测量模式"="水样测试", "数据类型"="N", "检测值"=0.0, "单位"="mg/L", "数据标识"="N", "信号值"=0.0, "标样参考值"=0.0, "因子编码"="", "探头温度"=0.0, "LastTime"=timestamp(0 s since 1904-01-01)} ("data"), "时间"=w183, "测量模式"="水样测试", "数据类型"=w181, "检测值"=w172, "单位"="mg/L", "数据标识"="N" ("水样数据标识"), "信号值"=w171, "因子编码"="", "探头温度"=w170, "数据标识"=w169) -> (w175:T1)
                  n214 = call "data insert.vi"("data"=w175, "table in"="氨氮") -> ("error out"=w177:errorcluster)  [unwired: 9 in]
                  n215 = Unbundle By Name(w177) -> ("status"=w178:bool)
                  n216 = Not(x=w178) -> (.not. x?=w185:bool)
                }
              }
            }
            n217 = case shown="True" w78 {
              tunnel: w75 -> [_ w129]
              tunnel: w79 -> [_ w127]
              frame False {
              }
              frame True {
                n218 = for {
                  N: 10 -> [_]
                  tunnel: w129 -> [w142]
                  tunnel: w127 -> [w134]
                  stop <- w146 stop-if-true
                  n219 = Unbundle By Name(w134) -> ("测量值"=w133:sgl, "信号值"=w132:sgl, "温度测量值"=w131:sgl, "数据标识"=w130:string)
                  n220 = Get Date/Time In Seconds() -> (seconds since 1Jan1904=w144:timestamp)
                  n221 = Bundle By Name(cluster=T1 {"时间"=timestamp(0 s since 1904-01-01), "测量模式"="水样测试", "数据类型"="N", "检测值"=0.0, "单位"="mg/L", "数据标识"="N", "信号值"=0.0, "标样参考值"=0.0, "因子编码"="", "探头温度"=0.0, "LastTime"=timestamp(0 s since 1904-01-01)} ("data"), "时间"=w144, "测量模式"="水样测试", "数据类型"=w142, "检测值"=w133, "单位"="mg/L", "数据标识"="N" ("水样数据标识"), "信号值"=w132, "因子编码"="w01012", "探头温度"=w131, "数据标识"=w130) -> (w136:T1)
                  n222 = call "data insert.vi"("data"=w136, "table in"="悬浮物") -> ("error out"=w138:errorcluster)  [unwired: 9 in]
                  n223 = Unbundle By Name(w138) -> ("status"=w139:bool)
                  n224 = Not(x=w139) -> (.not. x?=w146:bool)
                }
              }
            }
            n225 = case shown="True" w105 {
              tunnel: w75 -> [_ w380]
              tunnel: w98 -> [_ w378]
              frame False {
              }
              frame True {
                n226 = global read "多参数全局变量.vi" "盐度显示"() -> (w377:T4)
                n227 = for {
                  N: 10 -> [_]
                  tunnel: w380 -> [w386]
                  tunnel: w378 -> [w398]
                  tunnel: w377 -> [w385]
                  stop <- w403 stop-if-true
                  n228 = Unbundle By Name(w385) -> ("测量值"=w387:sgl, "温度测量值"=w388:sgl, "信号值"=w391:sgl, "数据标识"=w394:string)
                  n229 = Unbundle By Name(w398) -> ("测量值"=w407:sgl, "温度测量值"=w406:sgl, "信号值"=w401:sgl, "数据标识"=w397:string)
                  n230 = Get Date/Time In Seconds() -> (seconds since 1Jan1904=w390:timestamp)
                  n231 = Get Date/Time In Seconds() -> (seconds since 1Jan1904=w402:timestamp)
                  n232 = Bundle By Name(cluster=T1 {"时间"=timestamp(0 s since 1904-01-01), "测量模式"="水样测试", "数据类型"="N", "检测值"=0.0, "单位"="mg/L", "数据标识"="N", "信号值"=0.0, "标样参考值"=0.0, "因子编码"="", "探头温度"=0.0, "LastTime"=timestamp(0 s since 1904-01-01)} ("data"), "因子编码"="", "单位"="ppt", "时间"=w390, "检测值"=w387, "探头温度"=w388, "信号值"=w391, "测量模式"="水样测试", "数据类型"=w386, "数据标识"=w394) -> (w393:T1)
                  n233 = Bundle By Name(cluster=T1 {"时间"=timestamp(0 s since 1904-01-01), "测量模式"="水样测试", "数据类型"="N", "检测值"=0.0, "单位"="mg/L", "数据标识"="N", "信号值"=0.0, "标样参考值"=0.0, "因子编码"="", "探头温度"=0.0, "LastTime"=timestamp(0 s since 1904-01-01)} ("data"), "因子编码"="电导率", "单位"="μS/cm", "时间"=w402, "检测值"=w407, "探头温度"=w406, "信号值"=w401, "测量模式"="水样测试", "数据类型"=w386, "数据标识"=w397) -> (w399:T1)
                  n234 = call "data insert.vi"("data"=w399, "table in"="电导率" ("table输入")) -> ("error out"=w382:errorcluster)  [unwired: 9 in]
                  n235 = call "data insert.vi"("error in (no error)"=w382, "data"=w393, "table in"="盐度") -> ("error out"=w381:errorcluster)  [unwired: 8 in]
                  n236 = Unbundle By Name(w381) -> ("status"=w405:bool)
                  n237 = Not(x=w405) -> (.not. x?=w403:bool)
                }
              }
            }
          }
        }
      }
      frame "结束" {
        w470 = u16 0 items=["空闲", "水样测试", "标样核查"] ("多参数运行状态")
        n238 = case shown="True" w466 {
          frame False {
          }
          frame True {
            n239 = call "操作日志.vi"("日志信息"="【水样测试】结束") -> ()  [unwired: 10 in, 1 out]
          }
        }
      }
    }
    "运行状态" <- w31
    n240 = Format Into String(format string=w39, w25) -> (resulting string=→"多参数运行日志":string)  [unwired: 2 in, 1 out]
    n241 = global write "多参数全局变量.vi" "多参数运行状态"(w31) -> ()
  }
